vi "Set OP and Post OP Measurements.vi"(8 "error in (no error)":errorcluster, 11 "Harmonics in":refnum<class "Harmonics.lvclass">) -> (0 "error out":errorcluster, 3 "Harmonics out":refnum<class "Harmonics.lvclass">)   [LabVIEW 2016]
uses:
  Plugins/QPA Measurement.lvlibp/QPA Measurement.lvclass
  C:/Sequence Automation/Plugins/Measurement Interface.lvlibp/Measurement Interface.lvclass
  C:/Sequence Automation/Plugins/FPF.lvlibp/Factory Plugin Framework.lvclass
  Harmonics.lvclass
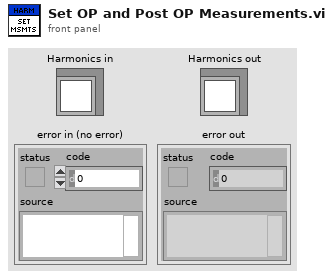
[diagram p1: front panel]
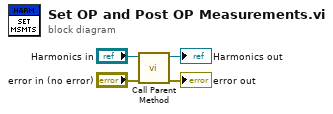
[diagram p0: block diagram]
diagram:
  n1 = call-parent "Call Parent Method"("error in (no error)"="error in (no error)", "QPA Measurement in"="Harmonics in") -> ("error out"=→"error out":errorcluster, "QPA Measurement out"=→"Harmonics out":refnum<class "QPA Measurement.lvclass">)  [unwired: 8 in]
